vi "Register for Events.vi"(8 "error in (no error)":errorcluster, 11 "eActor in":refnum<class "eActor.lvclass">) -> (0 "error out":errorcluster, 2 "Event Registration Refnum":variant, 3 "eActor out":refnum<class "eActor.lvclass">)   [LabVIEW 2015, in "AMS UI.lvlib" / "eActor.lvclass"]
uses:
  eActor.lvclass
  eActor.lvclass/eActor.ctl
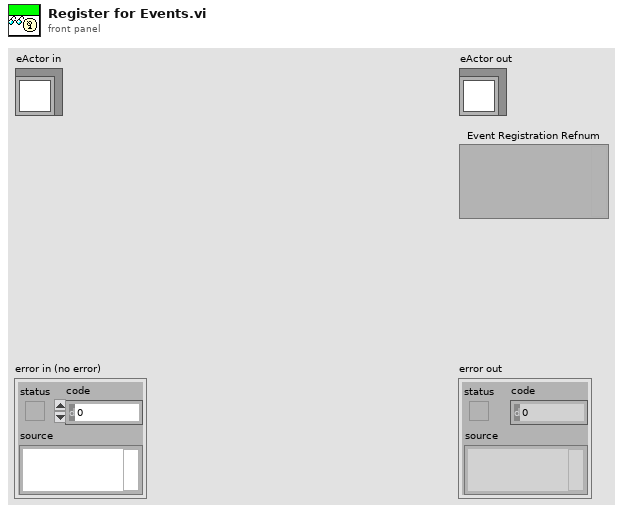
[diagram p1: front panel]
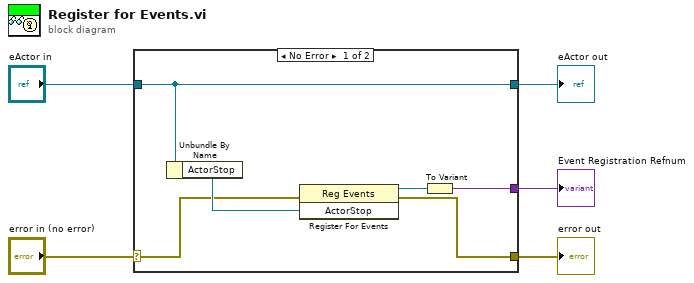
[diagram p0: block diagram]
diagram:
  n1 = case shown="No Error" "error in (no error)" {
    selector: "error in (no error)" -> [w8 w12]
    tunnel: [w7 w12] -> w4
    tunnel: [w11 w13] -> w2
    tunnel: "eActor in" -> [w11 w13]
    tunnel: [w6 _] -> w1
    frame No Error {
      n2 = Unbundle By Name(w11) -> ("ActorStop"=w10:refnum<user-event>)
      n3 = register-events(error in=w8, w10) -> (reference out=w9:refnum<event-registration>, error out=w7:errorcluster)  [unwired: 1 in]
      n4 = To Variant(anything=w9) -> (Variant=w6:variant)
    }
    frame Error {
    }
  }
  "error out" <- w4
  "eActor out" <- w2
  "Event Registration Refnum" <- w1
